vi "D_A Output Scale.vi"(7 "Read Value? (F)":bool, 8 "error in (no error)":errorcluster, 10 "Output Scale (Log)":T1, 11 "VISA resource name":refnum<visa-resource-name>) -> (0 "error out":errorcluster, 2 "Output Scale":T1, 3 "VISA resource name out":refnum<visa-resource-name>)   [LabVIEW 2013, in "SRS SR400.lvlib"]
doc: "<B>AM { j }</B>\n\nIf j is included, the AM command sets the D/A output scale. If j is absent, the D/A output scale is returned.\n\n<B>j</B> <B>Output scale</B>\n0 Log (1V/decade)\n1 987######\n2 #876#####\n3 ##765####\n4 ###654###\n5 ####543##\n6 #####432#\n7 ######321"
uses:
  <instrlib>/SRS SR400/SRS SR400.lvlib
  <instrlib>/SRS SR400/Public/Typedefs/Output Scale.ctl
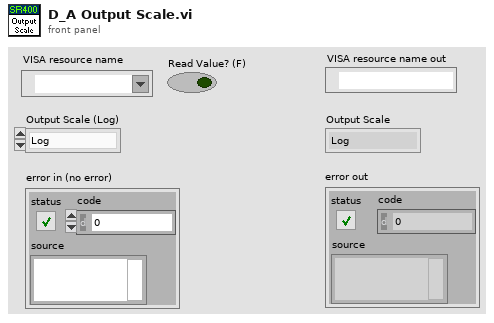
[diagram p1: front panel]
types:
  T1 = typedef "SRS SR400.lvlib/Output Scale.ctl" = enum16{"Log", "987######", "#876#####", "##765####", "###654###", "####543##", "#####432#", "######321"}
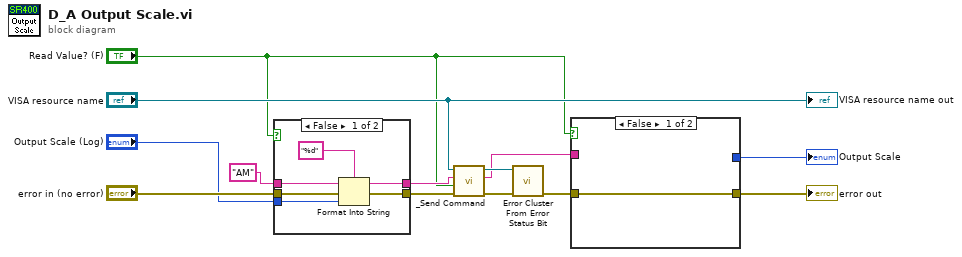
[diagram p0: block diagram]
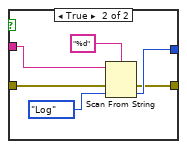
[diagram p2: hidden frame]
diagram:
  n1 = case shown="False" "Read Value? (F)" {
    tunnel: "error in (no error)" -> [w19 w20]
    tunnel: "AM" ("command") -> [w17 w21]
    tunnel: [w16 w21] -> w11
    tunnel: [w15 w20] -> w10
    tunnel: "Output Scale (Log)" -> [w14 _]
    frame False {
      n2 = Format Into String(format string="%d", initial string=w17, error in=w19, w14) -> (resulting string=w16:string, error out=w15:errorcluster)
    }
    frame True {
    }
  }
  n3 = call <instrlib>:"_Send Command.vi"("error in (no error)"=w10, "Read Value? (F)"="Read Value? (F)", "Command"=w11, "VISA resource name"="VISA resource name") -> ("error out"=w7:errorcluster, "Response"=w3:string, "VISA resource name out"=w6:refnum<visa-resource-name>)  [unwired: 5 out]
  n4 = call <instrlib>:"Error Cluster From Error Status Bit.vi"("error in (no error)"=w7, "VISA resource name"=w6) -> ("error out"=w4:errorcluster)  [unwired: 8 in, 1 out]
  n5 = case shown="False" "Read Value? (F)" {
    tunnel: w4 -> [w22 w28]
    tunnel: w3 -> [_ w26]
    tunnel: [_ w24] -> w2
    tunnel: [w22 w23] -> w1
    frame False {
    }
    frame True {
      n6 = Scan From String(format string="%d", input string=w26, error in=w28, default 1=Output_Scale."Log" ("Output Scale (Log)")) -> (error out=w23:errorcluster, output 1=w24:T1)  [unwired: 1 in, 2 out]
    }
  }
  "error out" <- w1
  "Output Scale" <- w2
  "VISA resource name out" <- "VISA resource name"
